vi "Run_Test.vi"(8 "error in (no error)":errorcluster caption="entrée d'erreur (pas d'erreur)", 11 "Test (Default) en entrée":refnum<class "Test (Default).lvclass">) -> (0 "error out":errorcluster caption="sortie d'erreur", 3 "Test (Default) en sortie":refnum<class "Test (Default).lvclass">)   [LabVIEW 2020, in "Library Test.lvlib" / "Test (Default).lvclass"]
uses:
  Test (Default).lvclass
  Test (Default).lvclass/Test (Default).ctl
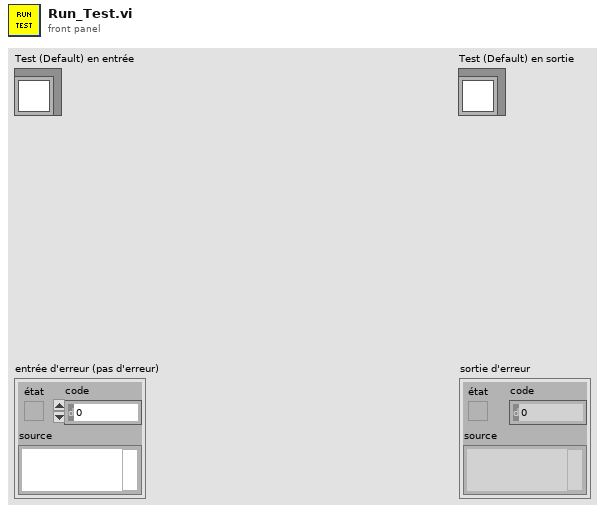
[diagram p1: front panel]
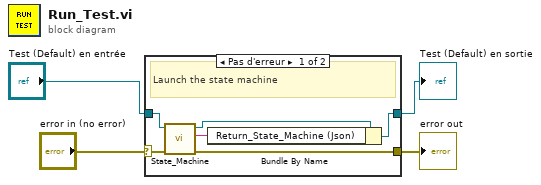
[diagram p0: block diagram]
diagram:
  n1 = case shown="Pas d'erreur" "error in (no error)" {
    selector: "error in (no error)" -> [w8 w12]
    tunnel: [w7 w12] -> w2
    tunnel: [w10 w11] -> w1
    tunnel: "Test (Default) en entrée" -> [w9 w11]
    frame No Error {
      # "Launch the state machine"
      n2 = call-dynamic "State_Machine.vi"("error in (no error)"=w8, "Test (Default) en entrée"=w9) -> ("error out"=w7:errorcluster, "Json_String"=w5:string, "Test (Default) en sortie"=w6:refnum<class "Test (Default).lvclass">)  [unwired: 7 in]
      n3 = Bundle By Name(cluster=w6, "Return_State_Machine (Json)"=w5) -> (w10:refnum<class "Test (Default).lvclass">)
    }
    frame Error {
    }
  }
  "error out" <- w2
  "Test (Default) en sortie" <- w1
